vi "Auto Iterate.vi"() -> (2 "Msg Strategy":refnum<class "Msg Strategy.lvclass">)   [LabVIEW 2021, in "Hello World Event.lvlib" / "Auto Iterate Msg Strategy.lvlib"]
uses:
  Auto Iterate Msg Strategy.lvlib
  <vilib>/Nathan Davis/jettl/jettl/Msg Strategy/Msg Strategy.lvclass
  Auto Iterate Msg Strategy/Auto Iterate Msg Strategy.lvclass
  C:/Program Files/National Instruments/LabVIEW 2021/vi.lib/Nathan Davis/jettl/jettl/Msg Strategy/Msg Strategy.lvclass
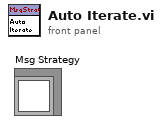
[diagram p1: front panel]
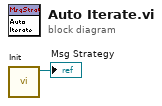
[diagram p0: block diagram]
diagram:
  n1 = call "Init.vi"() -> ("Auto Iterate Msg Strategy out"=→"Msg Strategy":refnum<class "Auto Iterate Msg Strategy.lvclass">)  [unwired: 11 in]
